vi "Move Absolute.vi"(4 "error in (no error)":errorcluster, 5 "Position (0 units)":dbl min=-2000000000.0 max=2000000000.0 format="%.6f", 6 "Axis (1)":i32=1 min=1 max=3, 7 "VISA resource name":refnum<visa-resource-name>) -> (0 "error out":errorcluster, 3 "VISA resource name out":refnum<visa-resource-name>)   [LabVIEW 2020, in "Newport ESP301.lvlib"]
doc: "This command initiates an absolute motion. When received, the selected axis <B>Axis (1)</B> will move, with the predefined acceleration and velocity, to the absolute position specified by <B>Position (0 units)</B>. If the requested axis is member of a group, this command does not initiate the desired motion. Instead, error xx31, \" COMMAND NOT ALLOWED DUE TO GROUP ASSIGNMENT\" is generated. Refer HL and HC commands to move along a line or an arc.\nIf this command is issued when trajectory mode for this axis is not in trapezoidal or s-curve mode, the controller returns error xx32, “INVALID TRAJECTORY MODE FOR MOVING”.\n<B>NOTE:</B> Even though the command is accepted while a motion is in progress, care should be taken not to reverse direction of motion. When this command is received, the controller verifies if it will produce a change of direction."
uses:
  Newport ESP301.lvlib
panel:
  out "decimal integer string":string
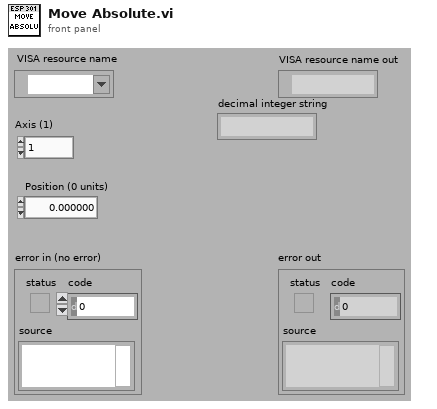
[diagram p1: front panel]
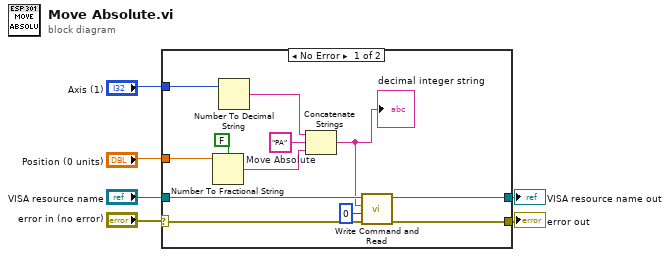
[diagram p0: block diagram]
diagram:
  n1 = case shown="No Error" "error in (no error)" {
    selector: "error in (no error)" -> [w15 w20]
    tunnel: [w17 w20] -> w6
    tunnel: "VISA resource name" -> [w18 w19]
    tunnel: [w16 w19] -> w5
    tunnel: "Axis (1)" -> [w11 _]
    tunnel: "Position (0 units)" -> [w10 _]
    frame No Error {
      w14 = "PA"  # Move Absolute
      n2 = Number To Fractional String(use system decimal point (T)=FALSE ("utiliser le séparateur décimal du système (V)"), number=w10) -> (F-format string=w13:string)  [unwired: 2 in]
      n3 = Number To Decimal String(number=w11) -> (decimal integer string=w12:string)  [unwired: 1 in]
      n4 = Concatenate Strings(w12, w14, w13) -> (w7:string)
      "decimal integer string" <- w7
      n5 = call "Write Command and Read.vi"("error in (no error)"=w15, "Bytes to read (100)"=u32 0, "Command"=w7, "VISA resource name"=w18) -> ("error out"=w17:errorcluster, "VISA resource name out"=w16:refnum<visa-resource-name>)  [unwired: 3 in, 1 out]
    }
    frame Error {
    }
  }
  "error out" <- w6
  "VISA resource name out" <- w5
